vi "moveSnake_subVI.vi"(5 "Old Direction Y":i32, 7 "Old Direction X":i32, 8 "New Direction X":i32, 9 "New Direction Y":i32, 10 "Snake Head X":i32, 11 "Snake Head Y":i32) -> (0 "New Snake Head X":i32, 1 "New Snake Head Y":i32, 2 "Current Direction X":i32, 3 "Current Direction Y":i32)   [LabVIEW 2020]
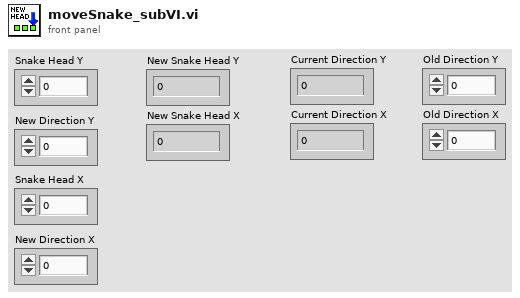
[diagram p1: front panel]
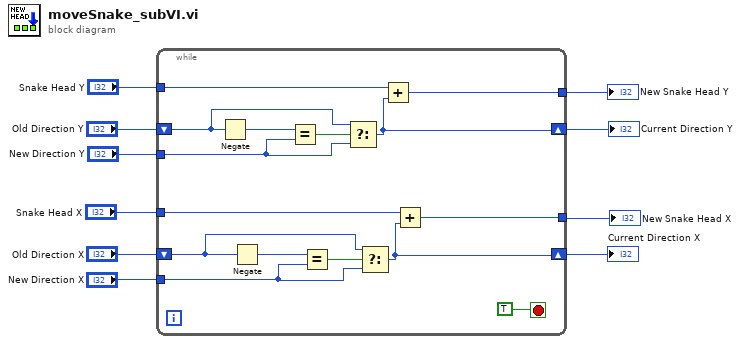
[diagram p0: block diagram]
diagram:
  n1 = while {
    tunnel: "Snake Head Y" -> [w24]
    tunnel: "New Direction Y" -> [w22]
    shift-right: [w21] -> w4
    shift-left: "Old Direction Y" -> [w19]
    tunnel: [w20] -> w6
    tunnel: [w16] -> w5
    tunnel: "Snake Head X" -> [w15]
    tunnel: "New Direction X" -> [w14]
    shift-right: [w12] -> w3
    shift-left: "Old Direction X" -> [w13]
    stop <- TRUE stop-if-true
    n2 = Negate(x=w19) -> (-x=w23:i32)
    n3 = Negate(x=w13) -> (-x=w18:i32)
    n4 = Equal?(x=w23, y=w22) -> (x = y?=w25:bool)
    n5 = Equal?(x=w18, y=w14) -> (x = y?=w17:bool)
    n6 = Select(t=w19, s=w25, f=w22) -> (s? t:f=w21:i32)
    n7 = Select(t=w13, s=w17, f=w14) -> (s? t:f=w12:i32)
    n8 = Add(x=w24, y=w21) -> (x+y=w20:i32)
    n9 = Add(x=w15, y=w12) -> (x+y=w16:i32)
  }
  "New Snake Head Y" <- w6
  "New Snake Head X" <- w5
  "Current Direction Y" <- w4
  "Current Direction X" <- w3
